vi "Generic file paths.vi"(8 "error in (no error)":errorcluster, 11 "Parent Folder":path=path "G:/My Drive/Nanosurf_data_processing/Nanosurf_data") -> (0 "error out":errorcluster, 3 "Paths":T1)   [LabVIEW 2016]
uses:
  Type-Defs/Paths.ctl
panel:
  out "result string":string
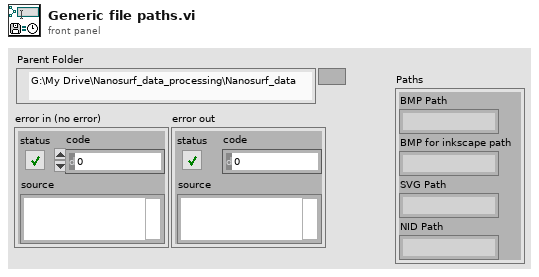
[diagram p1: front panel]
types:
  T1 = typedef "Paths.ctl" = cluster{"BMP Path":string, "BMP for inkscape path":string, "SVG Path":string, "NID Path":string}
  T2 = cluster{"BMP Path":string, "BMP for inkscape path":string, "SVG Path":string, "NID Path":string}
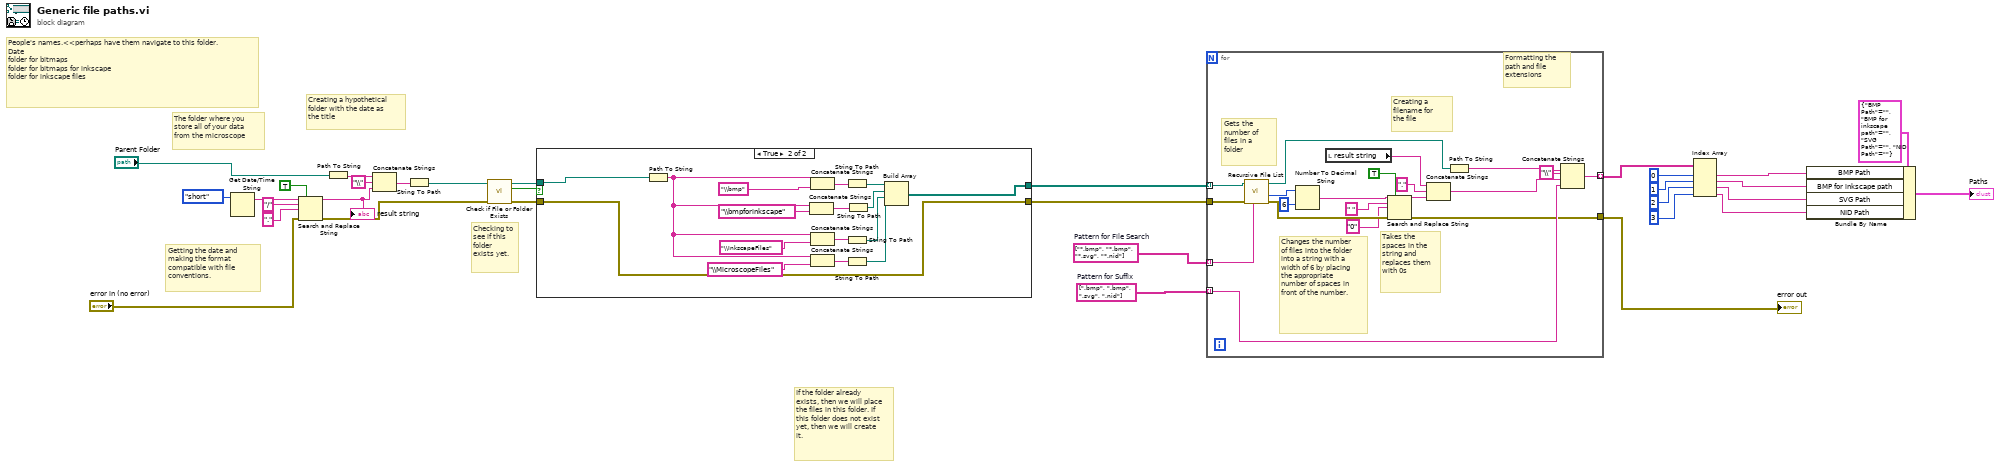
[diagram p0: block diagram]
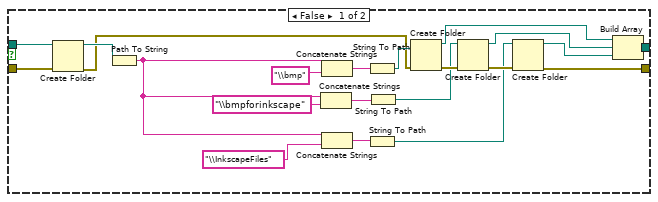
[diagram p2: hidden frame]
diagram:
  w13 = string[] ["*.bmp", "*.bmp", "*.svg", "*.nid"]  # Pattern for File Search
  w14 = string[] [".bmp", ".bmp", ".svg", ".nid"]  # Pattern for Suffix
  # "Checking to see if this folder exists yet."
  # "Creating a hypothetical folder with the date as the title"
  # "Getting the date and making the format compatible with file conventions."
  # "The folder where you store all of your data from the microscope"
  # "If the folder already exists, then we will place the files in this folder. If this folder does not exist yet, then we will create it."
  # "People's names.<<perhaps have them navigate to this folder.\nDate\nfolder for bitmaps\nfolder for bitmaps for inkscape\nfolder for inkscape files"
  n1 = Get Date/Time String(date format (0)=enum16{"short", "long", "abbreviated"}."short") -> (date string=w28:string)  [unwired: 2 in, 1 out]
  n2 = Search and Replace String(replace all?=TRUE ("replace all? (F)"), input string=w28, search string="/", replace string="." ("replace string (\"\")"), error in="error in (no error)") -> (result string=w19:string, error out=w21:errorcluster)  [unwired: 3 in, 2 out]
  "result string" <- w19
  n3 = Path To String(path="Parent Folder") -> (string=w25:string)
  n4 = Concatenate Strings(w25, "\\" ("string"), w19) -> (w23:string)
  n5 = String To Path(string=w23) -> (path=w22:path)
  n6 = call <vilib>:"Check if File or Folder Exists.vi"("error in (no error)"=w21, "path"=w22) -> ("error out"=w30:errorcluster, "file or folder exists?"=w31:bool, "dup path"=w32:path)  [unwired: 7 in]
  n7 = case shown="True" w31 {
    tunnel: w32 -> [w53 w62]
    tunnel: w30 -> [w52 w63]
    tunnel: [w41 w63] -> w20
    tunnel: [w33 w54] -> w15
    frame False {
      n8 = Create Folder(path (use dialog)=w53, error in=w52) -> (created path=w51:path, error out=w37:errorcluster)  [unwired: 1 in, 1 out]
      n9 = Path To String(path=w51) -> (string=w49:string)
      n10 = Concatenate Strings(w49, "\\bmpforinkscape" ("string")) -> (w45:string)
      n11 = Concatenate Strings(w49, "\\bmp" ("string")) -> (w46:string)
      n12 = Concatenate Strings(w49, "\\InkscapeFiles" ("string")) -> (w44:string)
      n13 = String To Path(string=w46) -> (path=w40:path)
      n14 = String To Path(string=w44) -> (path=w38:path)
      n15 = String To Path(string=w45) -> (path=w39:path)
      n16 = Create Folder(path (use dialog)=w40, error in=w37) -> (created path=w34:path, error out=w42:errorcluster)  [unwired: 1 in, 1 out]
      n17 = Create Folder(path (use dialog)=w39, error in=w42) -> (created path=w36:path, error out=w43:errorcluster)  [unwired: 1 in, 1 out]
      n18 = Create Folder(path (use dialog)=w38, error in=w43) -> (created path=w35:path, error out=w41:errorcluster)  [unwired: 1 in, 1 out]
      n19 = Build Array(w34, w36, w35) -> (w33:path[])
    }
    frame True {
      n20 = Path To String(path=w62) -> (string=w56:string)
      n21 = Concatenate Strings(w56, "\\bmpforinkscape" ("string")) -> (w65:string)
      n22 = Concatenate Strings(w56, "\\bmp" ("string")) -> (w66:string)
      n23 = Concatenate Strings(w56, "\\InkscapeFiles" ("string")) -> (w64:string)
      n24 = Concatenate Strings(w56, "\\MicroscopeFiles" ("string")) -> (w58:string)
      n25 = String To Path(string=w66) -> (path=w61:path)
      n26 = String To Path(string=w64) -> (path=w59:path)
      n27 = String To Path(string=w58) -> (path=w55:path)
      n28 = String To Path(string=w65) -> (path=w60:path)
      n29 = Build Array(w61, w60, w59, w55) -> (w54:path[])
    }
  }
  n30 = for {
    tunnel: w20 -> [w89]
    tunnel: w15 -> [w75] mode=indexing
    tunnel: w14 -> [w73] mode=indexing
    tunnel: [w72] -> w12 mode=indexing
    tunnel: w13 -> [w71] mode=indexing
    tunnel: [w70] -> w8
    # "Formatting the path and file extensions"
    # "Creating a filename for the file"
    # "Takes the spaces in the string and replaces them with 0s"
    # "Changes the number of files into the folder into a string with a width of 6 by placing the appropriate number of spaces in front of the number."
    # "Gets the number of files in a folder"
    n31 = call <vilib>:"Recursive File List.vi"("pattern"=w71, "error in (no error)"=w89, "Folder Path"=w75) -> ("error out"=w81:errorcluster, "Number of Files"=w78:i32, "dup Folder Path"=w79:path)  [unwired: 4 in, 2 out]
    n32 = Number To Decimal String(number=w78, width (-)=i16 6) -> (decimal integer string=w87:string)
    n33 = local read "result string"() -> (w82:string)
    n34 = Search and Replace String(replace all?=TRUE ("replace all? (F)"), input string=w87, search string=" ", replace string="0" ("replace string (\"\")"), error in=w81) -> (result string=w85:string, error out=w70:errorcluster)  [unwired: 3 in, 2 out]
    n35 = Concatenate Strings(w82, "." ("string"), w85) -> (w76:string)
    n36 = Path To String(path=w79) -> (string=w77:string)
    n37 = Concatenate Strings(w77, "\\" ("string"), w76, w73) -> (w72:string)
  }
  "error out" <- w8
  n38 = Index Array(array=w12, index #1=0 ("index"), index #2=1 ("index"), index #3=2 ("index"), index #4=3 ("index")) -> (element #1=w5:string, element #2=w4:string, element #3=w3:string, element #4=w2:string)
  n39 = Bundle By Name(cluster=T2 {"BMP Path"="", "BMP for inkscape path"="", "SVG Path"="", "NID Path"=""} ("Cluster"), "BMP Path"=w5, "BMP for inkscape path"=w4, "SVG Path"=w3, "NID Path"=w2) -> (→"Paths":T2)
